vi "kArrayBufferDblCirc.vi"(8 "HistLen":i32=1024, 11 "Input Vect":dbl[](array[numeric])=[0.0, 0.0]) -> (3 "Output Array":dbl[][](array[numeric]))   [LabVIEW 2010, in "kevLib2010.lvlib"]
uses:
  kevLib2010.lvlib
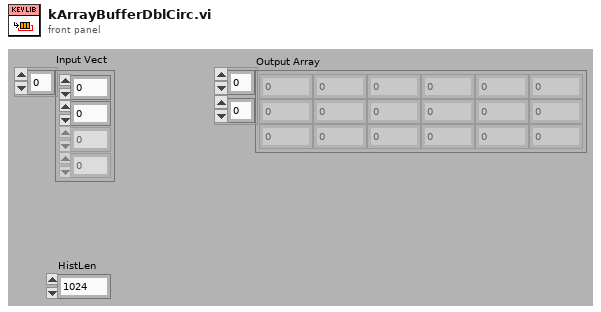
[diagram p1: front panel]
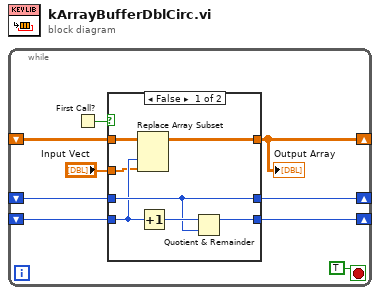
[diagram p0: block diagram]
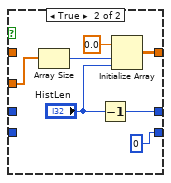
[diagram p2: hidden frame]
diagram:
  n1 = while {
    shift-right: [w2] -> _
    shift-left: _ -> [w7]
    shift-right: [w6] -> _
    shift-left: _ -> [w5]
    shift-right: [w4] -> _
    shift-left: _ -> [w3]
    stop <- TRUE stop-if-true
    n2 = First Call?() -> (First Call?: T/F=w9:bool)
    n3 = case shown="False" w9 {
      tunnel: "Input Vect" -> [w11 w22]
      tunnel: [w10 w20] -> w2
      tunnel: w7 -> [w13 _]
      tunnel: [w15 w18] -> w6
      tunnel: w5 -> [w15 _]
      tunnel: [w14 0 ("HistLen")] -> w4
      tunnel: w3 -> [w12 _]
      frame False {
        n4 = Replace Array Subset(array=w13, new element=w11, index (col)=w12) -> (w10:dbl[][])  [unwired: 1 in]
        n5 = Increment(x=w12) -> (x+1=w16:i32)
        n6 = Quotient & Remainder(x=w16, y=w15) -> (x-y*floor(x/y)=w14:i32)  [unwired: 1 out]
      }
      frame True {
        n7 = Array Size(array=w22) -> (size(s)=w21:i32)
        n8 = Decrement(x="HistLen") -> (x-1=w18:i32)
        n9 = Initialize Array(0.0 ("element"), w21, "HistLen") -> (w20:dbl[][])
      }
    }
    "Output Array" <- w2
  }
